vi "Quaternion_New.vi"(8 "Z":dbl, 9 "Y":dbl, 10 "X":dbl, 11 "W":dbl=1.0) -> (3 "out Quaternion":T1={"R"=1.0, "V"=[0.0, 0.0, 0.0]})   [LabVIEW 2019, in "Trajectory_Library.lvlib"]
doc: "Constructs a quaternion with using the provided inputs.\n\nParameters:\n -- w -- W component of the quaternion.\n -- x -- X component of the quaternion.\n -- y -- Y component of the quaternion.\n -- z -- Z component of the quaternion.\n \nReturns:\n - out Quaternion -- Created data cluster"
uses:
  Trajectory_Library.lvlib
  TypeDef/QUATERNION.ctl
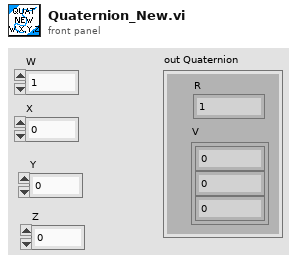
[diagram p1: front panel]
types:
  T1 = typedef "Trajectory_Library.lvlib/QUATERNION.ctl" = cluster{"R":dbl, "V":dbl[]}
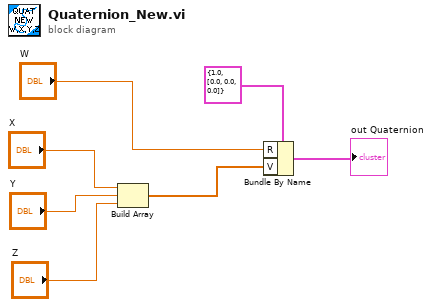
[diagram p0: block diagram]
diagram:
  n1 = Build Array("X", "Y", "Z") -> (w1:dbl[])
  n2 = Bundle By Name(cluster=T1 {"R"=1.0, "V"=[0.0, 0.0, 0.0]} ("sumPOSE"), "R"="W", "V"=w1) -> (→"out Quaternion":T1)
